vi "Modem Status Loop.vi"(1 "PCP IO Loop ID":u16, 11 "error in (no error)":errorcluster) -> ()   [LabVIEW 2011]
uses:
  Modem Status Raw Analog Data Cluster.ctl
  <vilib>/Instr/_visa.llb/VISA Flush IO Buffer Mask.ctl
  emi Lib/System 01/0 - General/App/Loop control 2/Private/_emi_ SMLoop start condition.vi
  emi Lib/System 01/0 - General/App/Loop control 2/Private/_emi_ SMLoop Error Check.vi
  emi Lib/Basic/0 - General/Error/emi_Is Error.vi
  emi Lib/System 01/0 - General/App/Loop control 2/Private/_emi_SMLoop Register new.vi
  emi Lib/System 01/0 - General/S&E reporting/emi_Send S&E Error message.vi
  emi Lib/Basic/0 - General/Error/emi_ Is Error state.vi
  emi Lib/System 01/0 - General/emi_Read System ID.vi
  emi Lib/System 01/0 - General/App/Loop control/Private/_emi_GFV Loop Linking.vi
  emi Lib/System 01/0 - General/App/Loop control/Private/_emi_GFV Loop Enable.vi
  emi Lib/System 01/0 - General/App/Loop control 2/Private/_emi_ SMLoop Restart.vi
  emi Lib/System 01/0 - General/App/Private/_emi_GFV App Close.vi
  emi Lib/System 01/0 - General/App/Loop control 2/Private/_emi_ SMLoop Restart Counter.vi
  emi Lib/System 01/0 - General/App/Loop control/Private/_emi_GFV Loop Running.vi
  emi Lib/System 01/0 - General/Private/_emi_GFV System ID.vi
  emi Lib/System 01/0 - General/S&E reporting/Private/_emi_S&E Q Generator.vi
  emi Lib/System 01/0 - General/App/Loop control/Private/_emi_GFV stop a loop so it can reset.vi
  <vilib>/Instr/_visa.llb/VISA Configure Serial Port (Instr).vi
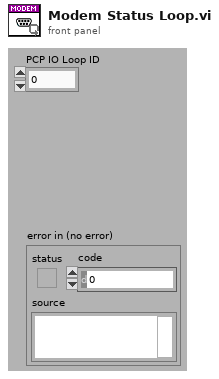
[diagram p1: front panel]
types:
  T1 = typedef "Modem Status Raw Analog Data Cluster.ctl" = cluster{"PCB Temp TS":dbl, "PCB Temp DH":dbl, "RX Gain TS":dbl, "RX Gain DH":dbl, "Signal Quality TS":dbl, "Signal Quality DH":dbl, "Numeric Link Status":dbl, "Link Status":bool}
  T2 = typedef "_emi_ SMLoop sates.ctl" = enum16{"Init", "Standby", "Start", "Normal Operation", "Stop", "Error Handling", "End", "Post"}
  T3 = cluster{"PCP cmd Q":refnum<queue>, "VISA name":refnum<visa-resource-name>, "Baud Rate":u32, "Address Table":u8[]}
  T4 = typedef "VISA Flush IO Buffer Mask.ctl" = u16
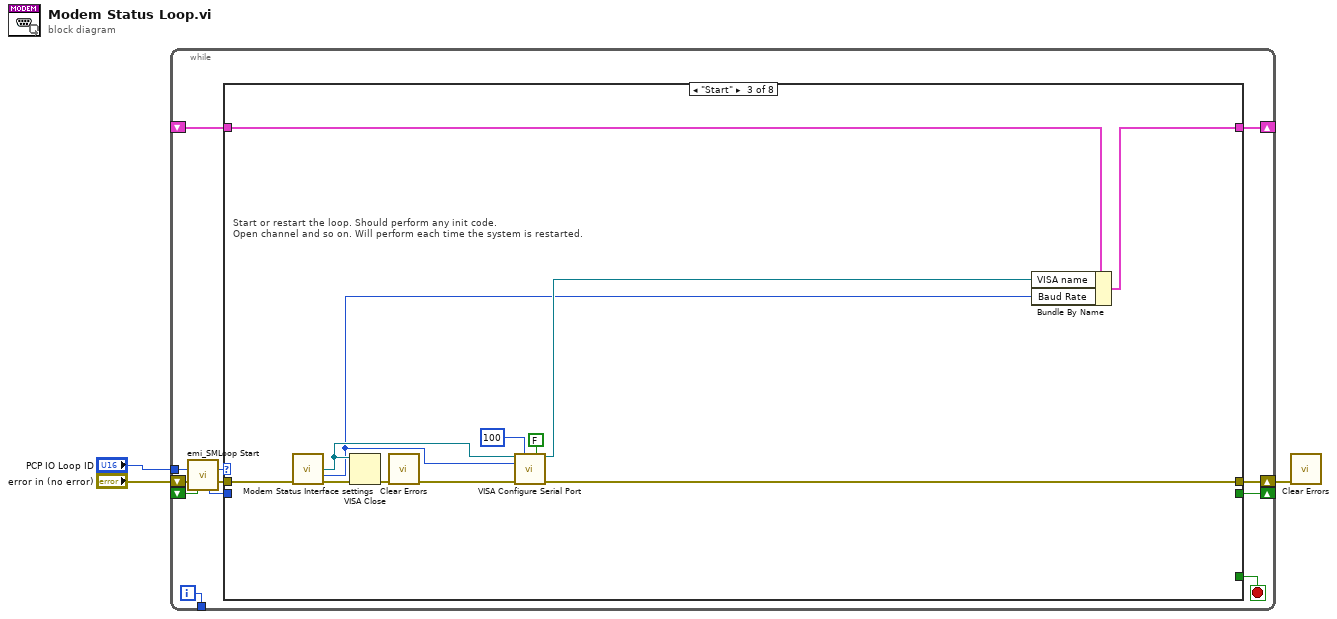
[diagram p0: block diagram]
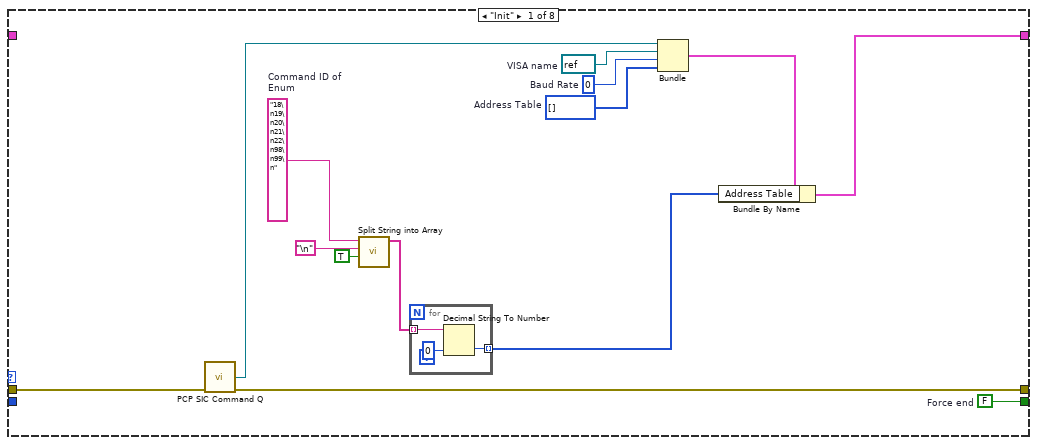
[diagram p2: hidden frame]
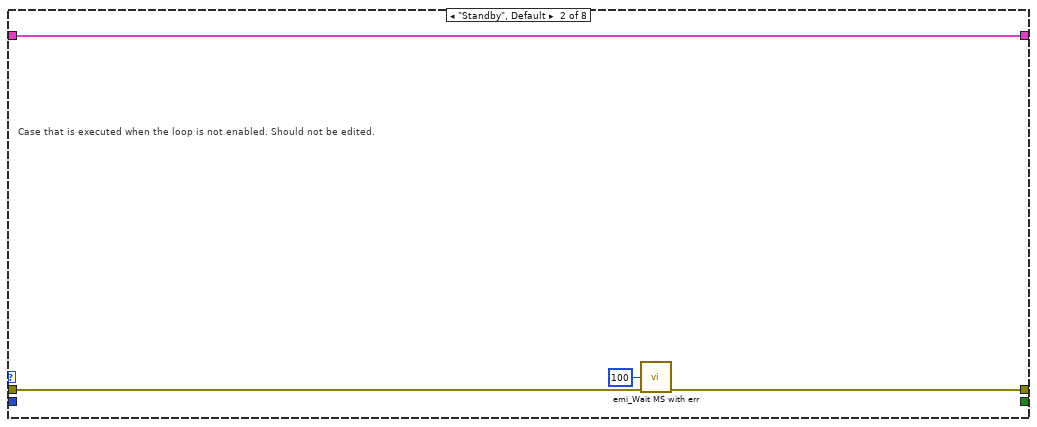
[diagram p3: hidden frame]
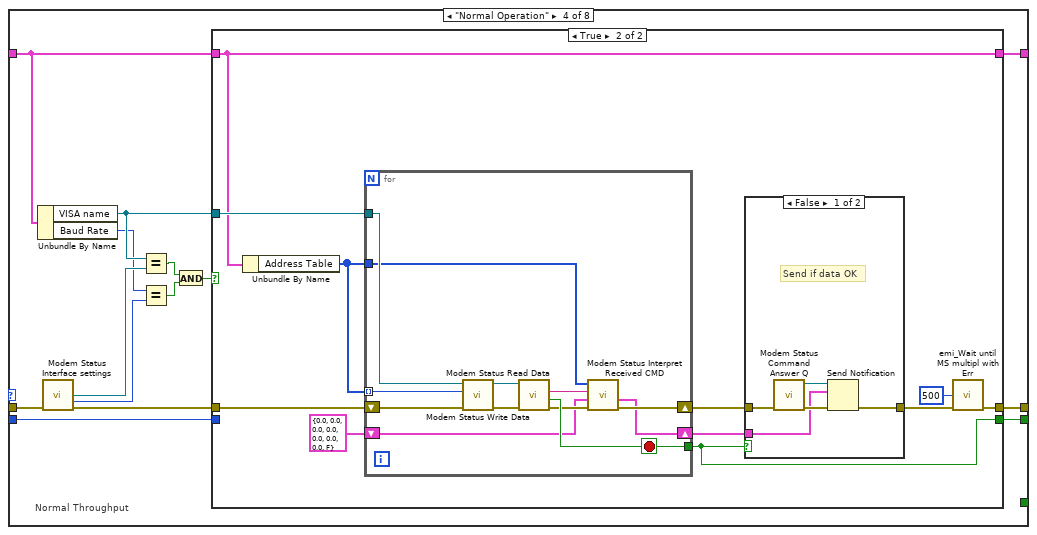
[diagram p4: hidden frame]
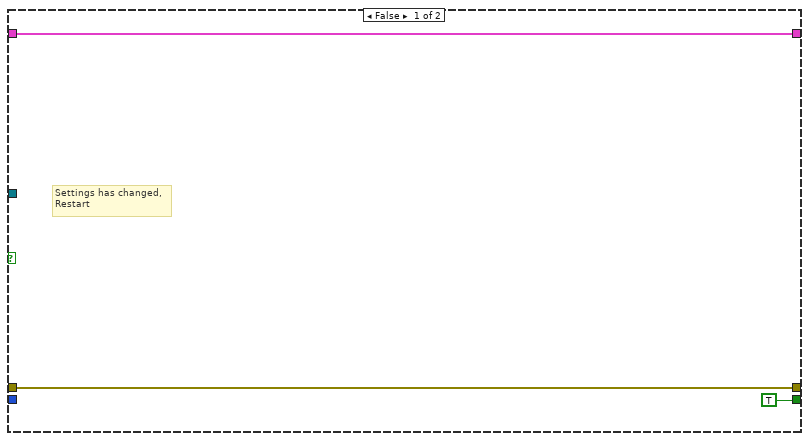
[diagram p5: hidden frame]
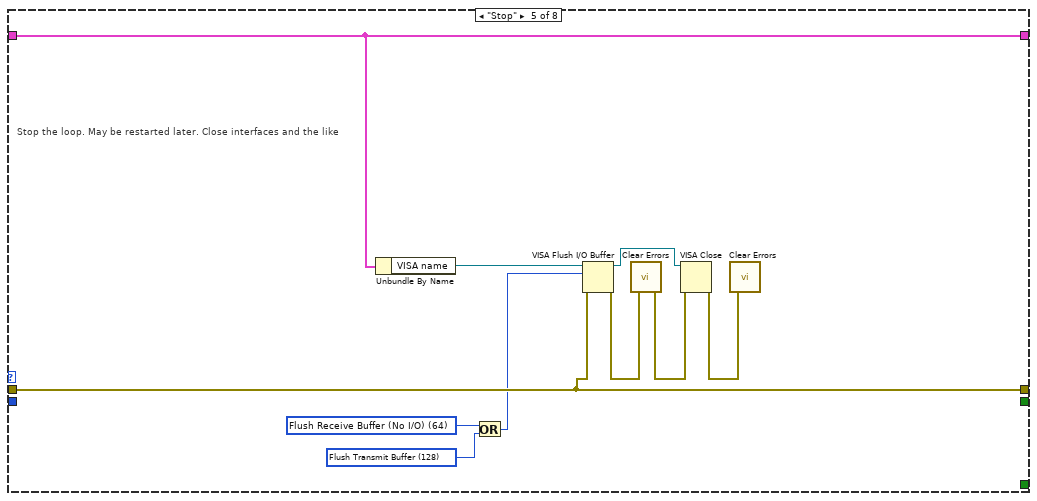
[diagram p7: hidden frame]
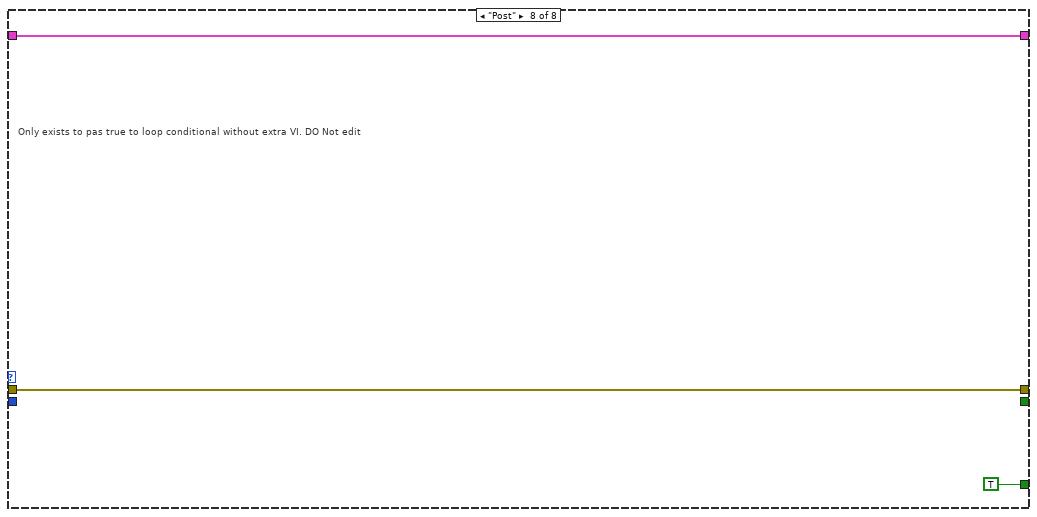
[diagram p10: hidden frame]
diagram:
  n1 = while {
    shift-right: [w15] -> _
    shift-left: _ -> [w11]
    shift-right: [w13] -> w1
    shift-left: "error in (no error)" -> [w9]
    tunnel: [w12] -> _
    shift-right: [w10] -> _
    shift-left: _ -> [w5]
    tunnel: "PCP IO Loop ID" -> [w6]
    i -> [w12]
    stop <- w14 stop-if-true
    n2 = call "emi_SMLoop Start.vi"("Loop ID"=w6, "error in (no error)"=w9, "Force Stop(F)"=w5) -> ("Loop command"=w7:T2, "error out"=w8:errorcluster, "Loop ID out"=w4:i32)  [unwired: 10 in]
    n3 = case shown="\"Start\"" w7 {
      tunnel: [w19 w33 w47 w61 w103 w106 w107 w110] -> w15
      tunnel: [_ _ _ _ _ _ _ TRUE] -> w14
      tunnel: w8 -> [w26 w35 w46 w56 w100 w105 w108 w111]
      tunnel: [w16 w34 w38 w62 w100 w105 w108 w111] -> w13
      tunnel: w11 -> [_ w33 w48 w60 w103 w106 w107 w110]
      tunnel: [w29 _ _ w59 _ _ _ _] -> w10
      tunnel: w4 -> [_ _ _ w58 _ _ _ _]
      frame "Init" {
        w18 = u8[] []  # Address Table
        w23 = "18\n19\n20\n21\n22\n98\n99\n"  # Command ID of  Enum
        w25 = u32 0  # Baud Rate
        w27 = refnum<visa-resource-name> refnum  # VISA name
        w29 = FALSE  # Force end
        n4 = call "PCP SIC Command Q.vi"("error in (no error)"=w26) -> ("PCP cmd Q"=w28:refnum<queue>, "error out"=w16:errorcluster)  [unwired: 13 in]
        n5 = call "Split String into Array.vi"("Remove Last Row"=TRUE, "Separator"="\n", "Input string"=w23) -> ("Array of cells"=w24:string[])  [unwired: 8 in]
        n6 = for {
          tunnel: w24 -> [w32] mode=indexing
          tunnel: [w30] -> w17 mode=indexing
          n7 = Decimal String To Number(string=w32, default (0L)=u8 0 ("default (0 I32)")) -> (number=w30:u8)  [unwired: 1 in, 1 out]
        }
        n8 = Bundle("PCP cmd Q"=w28, "VISA name"=w27, "Baud Rate"=w25, "Address Table"=w18) -> (w20:T3)  [unwired: 1 in]
        n9 = Bundle By Name(cluster=w20, "Address Table"=w17) -> (w19:T3)
      }
      frame "Standby", Default {
        # "Case that is executed when the loop is not enabled. Should not be edited."
        n10 = call "emi_Wait MS with err.vi"("milliseconds to wait(0)"=u32 100, "error in (no error)"=w35) -> ("error out"=w34:errorcluster)  [unwired: 13 in]
      }
      frame "Start" {
        # "Start or restart the loop. Should perform any init code. \nOpen channel and so on. Will perform each time the system is restarted."
        n11 = call "Modem Status Interface settings.vi"("error in (no error)"=w46) -> ("PCP VISA  name  out"=w42:refnum<visa-resource-name>, "baud rate out"=w37:u32, "error out"=w41:errorcluster)  [unwired: 12 in]
        n12 = VISA Close(VISA resource name=w42, error in (no error)=w41) -> (error out=w43:errorcluster)
        n13 = call <vilib>:"Clear Errors.vi"("error in (no error)"=w43) -> ("error out"=w40:errorcluster)  [unwired: 6 in]
        n14 = call-poly "VISA Configure Serial Port"("VISA resource name"=w42, "timeout (10sec)"=u32 100, "Enable Termination\nChar (T)"=FALSE ("Enable Termination\nChar (T)"), "baud rate (9600)"=w37, "error in (no error)"=w40) -> ("VISA resource name out"=w39:refnum<visa-resource-name>, "error out"=w38:errorcluster)  [unwired: 9 in]
        n15 = Bundle By Name(cluster=w48, "VISA name"=w39, "Baud Rate"=w37) -> (w47:T3)
      }
      frame "Normal Operation" {
        # "Normal Throughput"
        n16 = Unbundle By Name(w60) -> ("VISA name"=w57:refnum<visa-resource-name>, "Baud Rate"=w52:u32)
        n17 = call "Modem Status Interface settings.vi"("error in (no error)"=w56) -> ("PCP VISA  name  out"=w55:refnum<visa-resource-name>, "baud rate out"=w53:u32, "error out"=w54:errorcluster)  [unwired: 12 in]
        n18 = Equal?(x=w57, y=w55) -> (x = y?=w51:bool)
        n19 = Equal?(x=w52, y=w53) -> (x = y?=w50:bool)
        n20 = And(x=w51, y=w50) -> (x .and. y?=w49:bool)
        n21 = case shown="True" w49 {
          tunnel: w54 -> [w64 w74]
          tunnel: [w63 w72] -> w61
          tunnel: w60 -> [w63 w72]
          tunnel: [TRUE ("Force End") w70] -> w59
          tunnel: [w64 w76] -> w62
          tunnel: w57 -> [_ w73]
          tunnel: w58 -> [_ _]
          frame False {
            # "Settings has changed,\nRestart"
          }
          frame True {
            n22 = Unbundle By Name(w72) -> ("Address Table"=w66:u8[])
            n23 = for {
              tunnel: [w90] -> w70
              tunnel: w73 -> [w91]
              shift-right: [w86] -> w69
              shift-left: w74 -> [w93]
              tunnel: w66 -> [w89]
              shift-right: [w85] -> w68
              shift-left: T1 {"PCB Temp TS"=0.0, "PCB Temp DH"=0.0, "RX Gain TS"=0.0, "RX Gain DH"=0.0, "Signal Quality TS"=0.0, "Signal Quality DH"=0.0, "Numeric Link Status"=0.0, "Link Status"=FALSE} ("Modem Status Raw Analog Data Out") -> [w84]
              tunnel: w66 -> [w83] mode=indexing
              stop <- w90 stop-if-true
              n24 = call "Modem Status Write Data.vi"("error in (no error)"=w93, "CMD ID"=w83, "VISA Refnum in"=w91) -> ("error out"=w94:errorcluster, "VISA Refnum out"=w92:refnum<visa-resource-name>)  [unwired: 7 in]
              n25 = call "Modem Status Read Data.vi"("error in (no error)"=w94, "VISA Refnum in"=w92) -> ("error out"=w87:errorcluster, "Failed"=w90:bool, "Msg Body"=w88:string)  [unwired: 6 in, 1 out]
              n26 = call "Modem Status Interpret Received CMD.vi"("error in (no error)"=w87, "Modem Status Raw Analog Data"=w84, "Msg Body"=w88, "Address Table"=w89) -> ("error out"=w86:errorcluster, "Modem Status Raw Analog Data Out"=w85:T1)  [unwired: 6 in]
            }
            n27 = case shown="False" w70 {
              tunnel: w69 -> [w81 w82]
              tunnel: w68 -> [w77 _]
              tunnel: [w78 w82] -> w67
              frame False {
                # "Send if data OK"
                n28 = call "Modem Status Command Answer Q.vi"("error in (no error)"=w81) -> ("error out"=w79:errorcluster, "notifier out"=w80:refnum<notifier>)  [unwired: 9 in]
                n29 = Send Notification(notification=w77, notifier=w80, error in (no error)=w79) -> (error out=w78:errorcluster)  [unwired: 1 out]
              }
              frame True {
              }
            }
            n30 = call "emi_Wait until MS multipl with Err.vi"("millisecond multiple(0)"=u32 500 ("milliseconds to wait(0)"), "error in (no error)"=w67) -> ("error out"=w76:errorcluster)  [unwired: 13 in]
          }
        }
      }
      frame "Stop" {
        w95 = T4 128 items=["Flush Receive Buffer"=16, "Write Transmit Buffer to Device"=32, "Flush Receive Buffer (No I/O)"=64, "Flush Transmit Buffer"=128] ("Mask")
        w97 = T4 64 items=["Flush Receive Buffer"=16, "Write Transmit Buffer to Device"=32, "Flush Receive Buffer (No I/O)"=64, "Flush Transmit Buffer"=128] ("Mask")
        # "Stop the loop. May be restarted later. Close interfaces and the like"
        n31 = Unbundle By Name(w103) -> ("VISA name"=w99:refnum<visa-resource-name>)
        n32 = Or(x=w97, y=w95) -> (x .or. y?=w96:T4)
        n33 = VISA Flush I/O Buffer(VISA resource name=w99, mask (16)=w96, error in (no error)=w100) -> (VISA resource name out=w98:refnum<visa-resource-name>, error out=w101:errorcluster)
        n34 = call <vilib>:"Clear Errors.vi"("error in (no error)"=w101) -> ("error out"=w102:errorcluster)  [unwired: 6 in]
        n35 = VISA Close(VISA resource name=w98, error in (no error)=w102) -> (error out=w104:errorcluster)
        n36 = call <vilib>:"Clear Errors.vi"("error in (no error)"=w104) -> ()  [unwired: 6 in, 1 out]
      }
      frame "Error Handling" {
        # "Loop automaticaly returns here after error is found. If error is cleared, \nLoop wil continue as normal(if was operative when error."
      }
      frame "End" {
        # "Only executes at application end has. Should performa any action the loop \nneeds to finnish. Executes only once."
      }
      frame "Post" {
        # "Only exists to pas true to loop conditional without extra VI. DO Not edit"
      }
    }
  }
  n37 = call <vilib>:"Clear Errors.vi"("error in (no error)"=w1) -> ()  [unwired: 6 in, 1 out]
